vi "Set Control Position.vi"(8 "error in (no error)":errorcluster, 9 "Size":T2, 10 "Position":T1, 11 "Ctl Refnum":refnum<vi>) -> (0 "error out":errorcluster, 1 "Availible?":bool, 3 "refnum dub":refnum<vi>)   [LabVIEW 2009, in "POLARIS Vision utility.lvlib"]
uses:
  POLARIS Vision utility.lvlib
  <vilib>/Utility/miscctls.llb/LVBoundsTypeDef.ctl
  <vilib>/Utility/miscctls.llb/LVPositionTypeDef.ctl
  XDisplay/POLARIS IMAQ Display.xctl
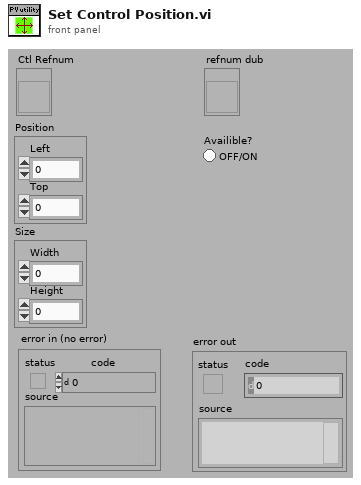
[diagram p1: front panel]
types:
  T1 = typedef "LVPositionTypeDef.ctl" = cluster{"Left":i32, "Top":i32}
  T2 = typedef "LVBoundsTypeDef.ctl" = cluster{"Width":u32, "Height":u32}
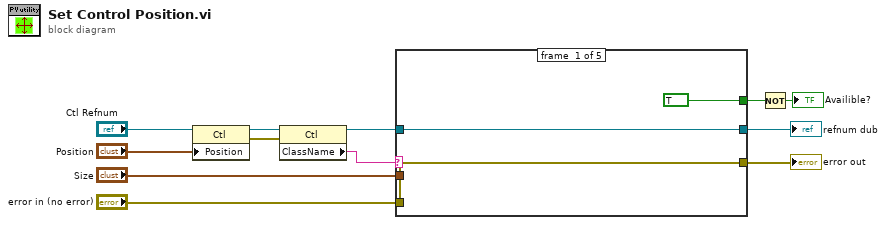
[diagram p0: block diagram]
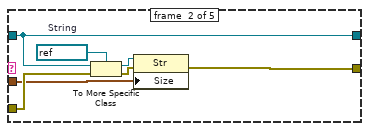
[diagram p2: hidden frame]
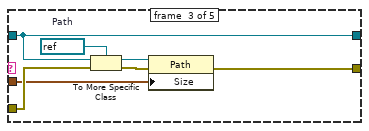
[diagram p3: hidden frame]
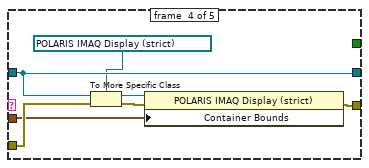
[diagram p4: hidden frame]
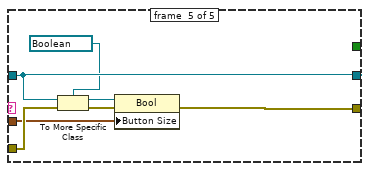
[diagram p5: hidden frame]
diagram:
  n1 = property class="Ctl"(reference="Ctl Refnum", "Position"="Position") -> (reference out=w2:refnum<vi>, error out=w3:errorcluster)  [unwired: 1 in]
  n2 = property class="Ctl"(reference=w2, error in=w3) -> (reference out=w1:refnum<vi>, "ClassName"=w5:string)  [unwired: 1 out]
  n3 = case shown="\"Boolean\"" w5 {
    tunnel: [w15 w17 w24 w35 w39] -> w12
    tunnel: w1 -> [w15 w17 w24 w35 w39]
    tunnel: "error in (no error)" -> [w14 w20 w27 w34 w42]
    tunnel: [w14 w18 w25 w32 w40] -> w10
    tunnel: [TRUE _ _ _ _] -> w9
    tunnel: "Size" -> [_ w16 w23 w30 w38]
    frame #0 {
    }
    frame #1 {
      w21 = refnum<vi> refnum  # String
      n4 = To More Specific Class(target class=w21, reference=w17, error in=w20) -> (specific class reference=w22:refnum<vi>, error out=w19:errorcluster)
      n5 = property class="Str"(reference=w22, error in=w19, "Size"=w16) -> (error out=w18:errorcluster)  [unwired: 1 out]
    }
    frame #2 {
      w28 = refnum<vi> refnum  # Path
      n6 = To More Specific Class(target class=w28, reference=w24, error in=w27) -> (specific class reference=w29:refnum<vi>, error out=w26:errorcluster)
      n7 = property class="Path"(reference=w29, error in=w26, "Size"=w23) -> (error out=w25:errorcluster)  [unwired: 1 out]
    }
    frame #3 {
      n8 = To More Specific Class(target class=refnum<vi> refnum ("POLARIS IMAQ"), reference=w35, error in=w34) -> (specific class reference=w36:refnum<vi>, error out=w33:errorcluster)
      n9 = property class="POLARIS IMAQ Display (strict)"(reference=w36, error in=w33, "Container Bounds"=w30) -> (error out=w32:errorcluster)  [unwired: 1 out]
    }
    frame #4 {
      n10 = To More Specific Class(target class=refnum<vi> refnum ("Bool Refnum"), reference=w39, error in=w42) -> (specific class reference=w43:refnum<vi>, error out=w41:errorcluster)
      n11 = property class="Bool"(reference=w43, error in=w41, "Button Size"=w38) -> (error out=w40:errorcluster)  [unwired: 1 out]
    }
  }
  "refnum dub" <- w12
  "error out" <- w10
  n12 = Not(x=w9) -> (.not. x?=→"Availible?":bool)
